vi "CoboltLaser_ComPortWrite.vi"(0 "ComPort":refnum<visa-resource-name>, 1 "Command":string, 2 "Data":string, 3 "ResponseWaitTime (s)":dbl=0.5 min=0.0 max=100.0 step=0.1, 5 "error in (no error)":errorcluster) -> (14 "ComPortOut":refnum<visa-resource-name>, 19 "error out":errorcluster)   [LabVIEW 2012, in "Cobolt.lvclass"]
doc: "Use this template to build a VI to use as a subVI."
uses:
  Template/Cobolt.lvclass
  Instance           1 25Saved   PR59_ComPortWrite .vi
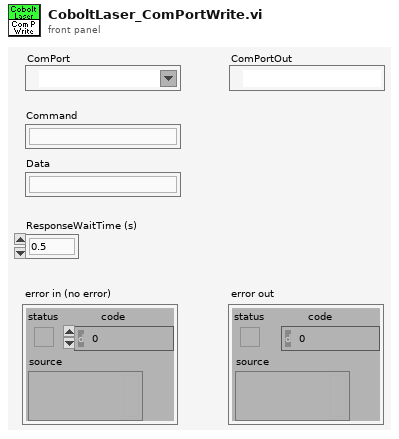
[diagram p1: front panel]
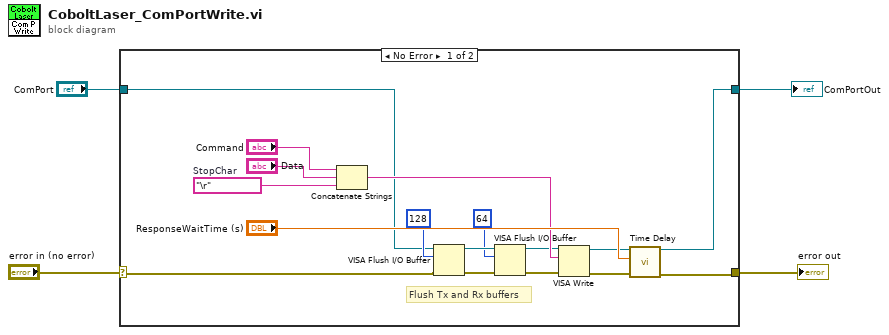
[diagram p0: block diagram]
diagram:
  n1 = case shown="No Error" "error in (no error)" {
    selector: "error in (no error)" -> [w12 w22]
    tunnel: [w18 w22] -> w3
    tunnel: "ComPort" -> [w6 w21]
    tunnel: [w5 w21] -> w1
    frame No Error {
      w7 = "\r"  # StopChar
      # "Flush Tx and Rx buffers"
      n2 = Concatenate Strings("Command", "Data", w7) -> (w17:string)
      n3 = VISA Flush I/O Buffer(VISA resource name=w6, mask (16)=u16 128, error in (no error)=w12) -> (VISA resource name out=w15:refnum<visa-resource-name>, error out=w16:errorcluster)
      n4 = VISA Flush I/O Buffer(VISA resource name=w15, mask (16)=u16 64, error in (no error)=w16) -> (VISA resource name out=w10:refnum<visa-resource-name>, error out=w11:errorcluster)
      n5 = VISA Write(VISA resource name=w10, write buffer=w17, error in (no error)=w11) -> (VISA resource name out=w5:refnum<visa-resource-name>, error out=w20:errorcluster)  [unwired: 1 out]
      n6 = call "Time Delay"("error in (no error)"=w20, "Delay Time (s)"="ResponseWaitTime (s)") -> ("error out"=w18:errorcluster)  [unwired: 9 out]
    }
    frame Error {
    }
  }
  "error out" <- w3
  "ComPortOut" <- w1
